vi "forceOutputState.vi"(8 "error in (no error)":errorcluster, 9 "calibratedValues":dbl[](array[numeric]), 10 "channel_addresses":string[](array[string]), 11 "niDAQmxDO in":refnum<class "niDAQmxDO.lvclass">) -> (0 "error out":errorcluster, 3 "niDAQmxDO out":refnum<class "niDAQmxDO.lvclass">)   [LabVIEW 2011, in "Hardware.lvlib" / "Channels.lvlib" / "niDAQmxDO.lvclass"]
uses:
  niDAQmxDO.lvclass
  <vilib>/DAQmx/write.llb/DAQmx Write (Digital 1D Wfm NChan NSamp).vi
  <vilib>/DAQmx/create/channels.llb/DAQmx Create Channel (DO-Digital Output).vi
  <vilib>/Waveform/DWDTOps.llb/DWDT Uncompress Digital.vi
  <vilib>/DAQmx/miscellaneous.llb/DAQmx Fill In Error Info.vi
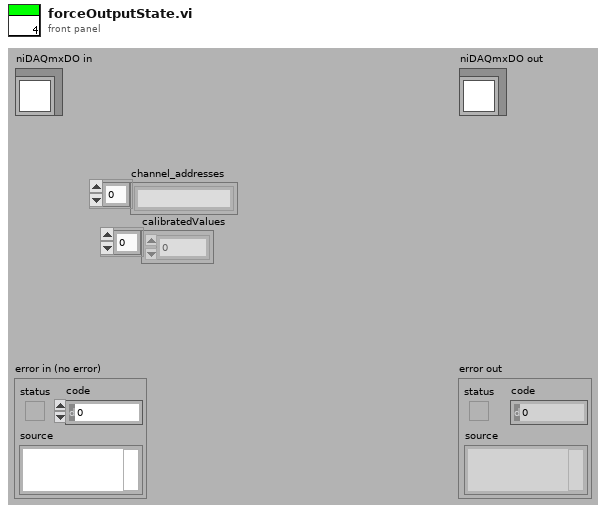
[diagram p1: front panel]
types:
  T1 = cluster{"Timestamps ms":dbl[], "Bitmap":bool[][]}
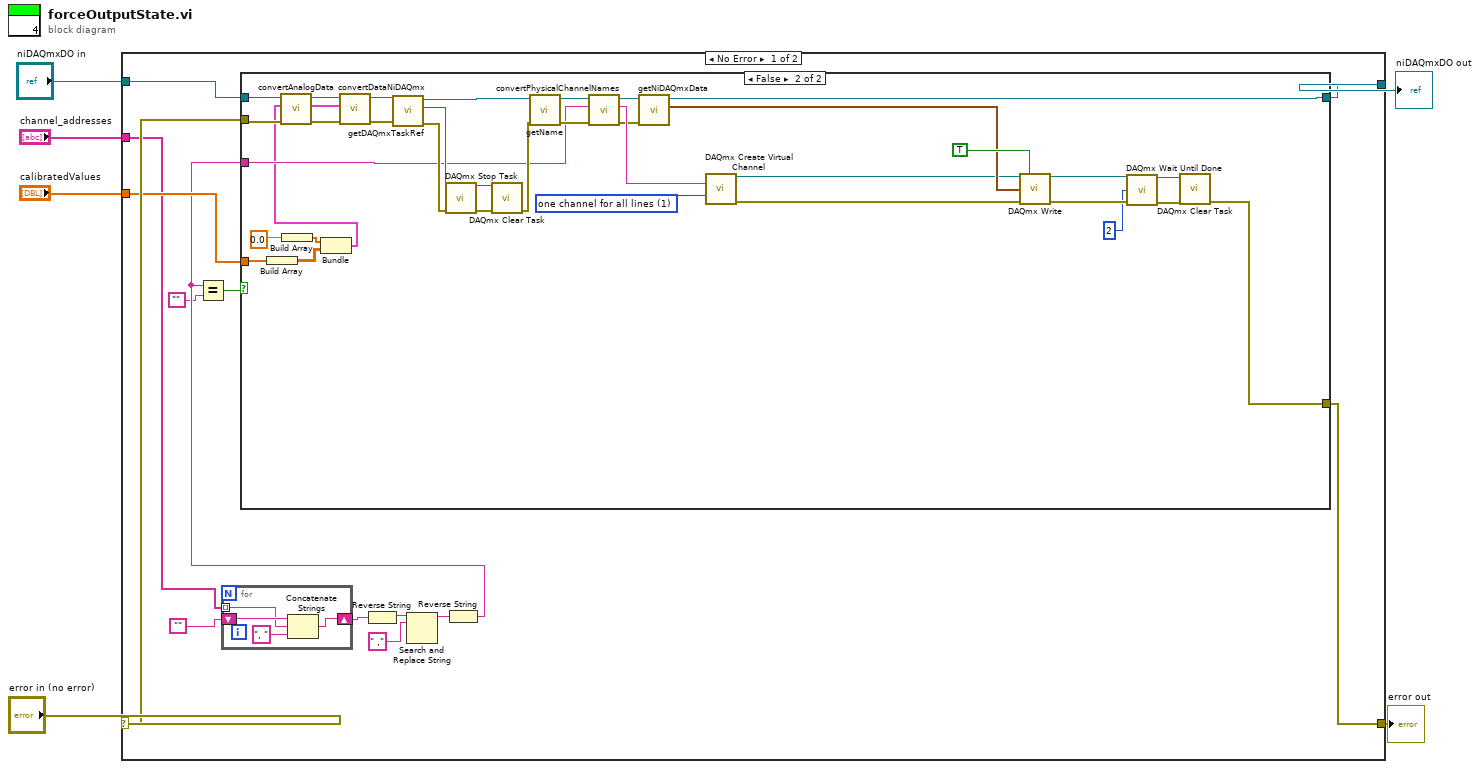
[diagram p0: block diagram]
diagram:
  n1 = case shown="No Error" "error in (no error)" {
    selector: "error in (no error)" -> [w19 w63]
    tunnel: [w8 w63] -> w5
    tunnel: [w7 w64] -> w3
    tunnel: "niDAQmxDO in" -> [w20 w64]
    tunnel: "channel_addresses" -> [w12 _]
    tunnel: "calibratedValues" -> [w18 _]
    frame No Error {
      n2 = for {
        tunnel: w12 -> [w23] mode=indexing
        shift-right: [w21] -> w16
        shift-left: "" -> [w24]
        n3 = Concatenate Strings(w24, w23, ", ") -> (w21:string)
      }
      n4 = Reverse String(1:w16) -> (0:w15:string)
      n5 = Search and Replace String(input string=w15, search string=" ,") -> (result string=w13:string)  [unwired: 6 in, 3 out]
      n6 = Reverse String(1:w13) -> (0:w10:string)
      n7 = Equal?(x=w10, y="") -> (x = y?=w11:bool)
      n8 = case shown="False" w11 {
        tunnel: w10 -> [_ w46]
        tunnel: w19 -> [w25 w43]
        tunnel: [w25 w55] -> w8
        tunnel: w20 -> [w26 w44]
        tunnel: [w26 w29] -> w7
        tunnel: w18 -> [_ w42]
        frame True {
        }
        frame False {
          w50 = 1 items=["one channel for each line", "one channel for all lines"] ("line grouping")
          n9 = Build Array(w42) -> (w40:dbl[][])
          n10 = Build Array(0.0) -> (w39:dbl[])
          n11 = Bundle(w39, w40) -> (w38:cluster{dbl[], dbl[][]})  [unwired: 1 in]
          n12 = call "convertAnalogData.vi"("error in (no error)"=w43, "Data"=w38, "niDAQmxDO in"=w44) -> ("error out"=w37:errorcluster, "digitalData"=w34:T1, "niDAQmxDO out"=w36:refnum<class "niDAQmxDO.lvclass">)  [unwired: 6 in]
          n13 = call "convertDataNiDAQmx.vi"("error in (no error)"=w37, "Data"=w34, "niDAQmxDO in"=w36) -> ("error out"=w33:errorcluster, "niDAQmxDO out"=w35:refnum<class "niDAQmxDO.lvclass">)  [unwired: 7 in]
          n14 = call "getDAQmxTaskRef.vi"("error in (no error)"=w33, "niDAQmxDO.lvclass in"=w35) -> ("error out"=w53:errorcluster, "DAQmx Task Ref"=w52:refnum<k21>, "niDAQmxDO.lvclass out"=w49:refnum<class "niDAQmxDO.lvclass">)  [unwired: 7 in]
          n15 = call <vilib>:"DAQmx Stop Task.vi"("task/channels in"=w52, "error in"=w53) -> ("task out"=w62:refnum<k21>, "error out"=w61:errorcluster)  [unwired: 12 in]
          n16 = call <vilib>:"DAQmx Clear Task.vi"("task in"=w62, "error in"=w61) -> ("error out"=w51:errorcluster)  [unwired: 13 in]
          n17 = call-dynamic "getName.vi"("error in (no error)"=w51, "DigitalOutput.lvclass in"=w49) -> ("error out"=w47:errorcluster, "DigitalOutput.lvclass out"=w48:refnum<class "niDAQmxDO.lvclass">)  [unwired: 7 in, 1 out]
          n18 = call "convertPhysicalChannelNames.vi"("error in (no error)"=w47, "PhysicalChannels"=w46, "niDAQmxDO in"=w48) -> ("error out"=w31:errorcluster, "channel_names"=w45:string, "niDAQmxDO out"=w32:refnum<class "niDAQmxDO.lvclass">)  [unwired: 6 in]
          n19 = call "getNiDAQmxData.vi"("error in (no error)"=w31, "niDAQmxDO.lvclass in"=w32) -> ("NIDAQmx data format"=w30:digitalwaveform[], "niDAQmxDO.lvclass out"=w29:refnum<class "niDAQmxDO.lvclass">)  [unwired: 7 in, 1 out]
          n20 = call-poly <vilib>:"DAQmx Create Virtual Channel.vi"("lines"=w45, "line grouping"=w50) -> ("task out"=w28:refnum<k21>, "error out"=w27:errorcluster)  [unwired: 12 in]
          n21 = call-poly <vilib>:"DAQmx Write.vi"("task/channels in"=w28, "auto start"=TRUE, "data"=w30, "error in"=w27) -> ("task out"=w59:refnum<k21>, "error out"=w58:errorcluster)  [unwired: 9 in, 1 out]
          n22 = call <vilib>:"DAQmx Wait Until Done.vi"("task/channels in"=w59, "timeout (sec)"=2, "error in"=w58) -> ("task out"=w57:refnum<k21>, "error out"=w56:errorcluster)  [unwired: 11 in]
          n23 = call <vilib>:"DAQmx Clear Task.vi"("task in"=w57, "error in"=w56) -> ("error out"=w55:errorcluster)  [unwired: 13 in]
        }
      }
    }
    frame Error {
    }
  }
  "error out" <- w5
  "niDAQmxDO out" <- w3
